vi "getTopicSubscriptions.vi"(8 "error in (no error)":errorcluster, 11 "SUBSCRIBE in":refnum<class "SUBSCRIBE.lvclass">) -> (0 "error out":errorcluster, 2 "Topic Subscriptions":T1[](array[typedef]), 3 "SUBSCRIBE out":refnum<class "SUBSCRIBE.lvclass">)   [LabVIEW 2013, in "SUBSCRIBE.lvclass"]
uses:
  SUBSCRIBE.lvclass
  Topic Subscription -- cluster.ctl
  ControlPacket/QualityOfService -- enum.ctl
  ControlPacket/ControlPacket.lvclass/ControlPacket.ctl
  ControlPacket/ControlPacket.lvclass
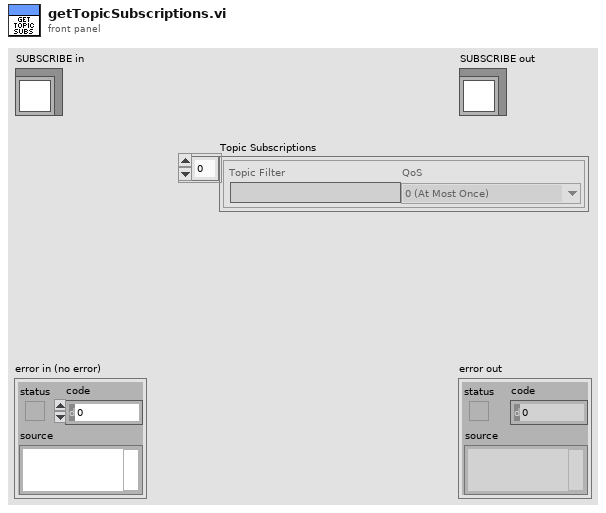
[diagram p1: front panel]
types:
  T1 = typedef "SUBSCRIBE.lvclass/Topic Subscription -- cluster.ctl" = cluster{"Topic Filter":string, "QoS":T2}
  T2 = typedef "ControlPacket.lvclass/QualityOfService -- enum.ctl" = enum16{"0 (At Most Once)", "1 (At Least Once)", "2 (Exactly Once)"}
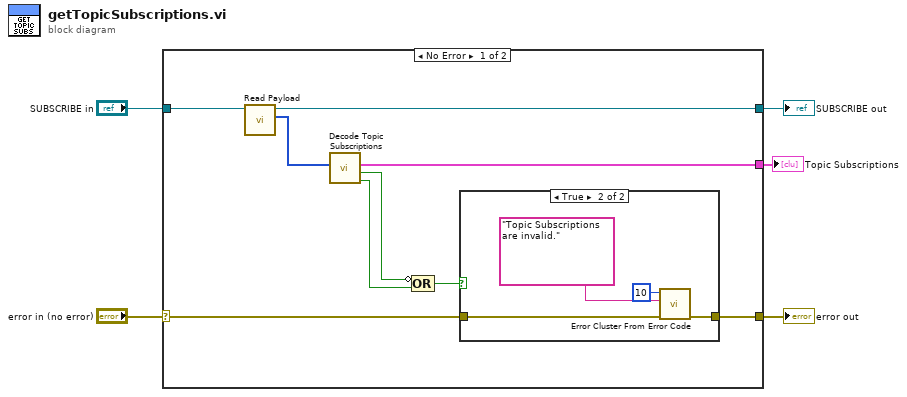
[diagram p0: block diagram]
diagram:
  n1 = case shown="No Error" "error in (no error)" {
    selector: "error in (no error)" -> [w10 w21]
    tunnel: [w9 w21] -> w4
    tunnel: [w13 w20] -> w2
    tunnel: "SUBSCRIBE in" -> [w14 w20]
    tunnel: [w11 _] -> w1
    frame No Error {
      n2 = call "Read Payload.vi"("ControlPacket in"=w14) -> ("Payload"=w12:u8[], "ControlPacket out"=w13:refnum<class "SUBSCRIBE.lvclass">)  [unwired: 9 in]
      n3 = call "Decode Topic Subscriptions.vi"("Payload"=w12) -> ("invalid UTF8"=w8:bool, "Valid?"=w7:bool, "Topic Subscriptions"=w11:T1[])  [unwired: 8 in]
      n4 = Compound Arithmetic op=OR(invert w7, w8) -> (w6:bool)
      n5 = case shown="True" w6 {
        tunnel: w10 -> [w15 w18]
        tunnel: [w15 w19] -> w9
        frame False {
        }
        frame True {
          n6 = call <vilib>:"Error Cluster From Error Code.vi"("error in (no error)"=w18, "error message (\"\")"="Topic Subscriptions are invalid." ("error source (\" \")"), "error code (0)"=10 ("error code (no error:0)")) -> ("error out"=w19:errorcluster)  [unwired: 6 in]
        }
      }
    }
    frame Error {
    }
  }
  "error out" <- w4
  "SUBSCRIBE out" <- w2
  "Topic Subscriptions" <- w1
